vi "poly_control_value_from_name_multi.vi"(8 "error in (no error)":errorcluster, 9 "control names":string[](array[string]), 10 "vi ref":refnum<vi>) -> (0 "error out":errorcluster, 1 "Values":variant[](array[variant]), 2 "vi ref dup":refnum<vi>, 4 "found?":bool[](array[boolean]), 5 "ctrl refs":refnum<vi>[](array[refnum]))   [LabVIEW 2015]
uses:
  poly_control_ref_from_name_multi.vi
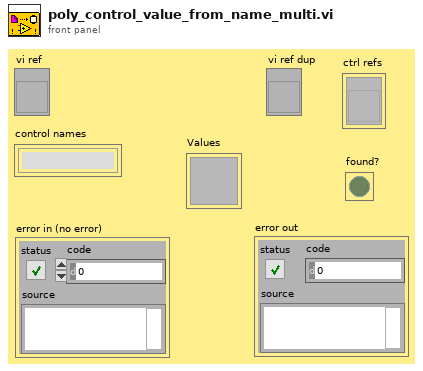
[diagram p1: front panel]
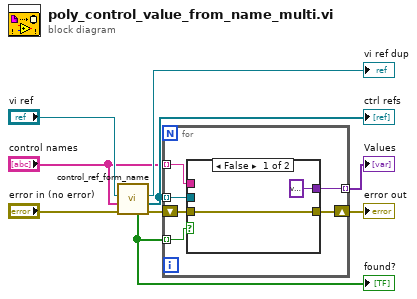
[diagram p0: block diagram]
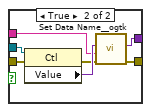
[diagram p2: hidden frame]
diagram:
  n1 = call-poly "control_ref_form_name.vi"("error in (no error)"="error in (no error)", "control names"="control names", "vi ref"="vi ref") -> ("error out"=w6:errorcluster, "ctrl refs"=w2:refnum<vi>[], "vi ref dup"=→"vi ref dup":refnum<vi>, "found?"=w3:bool[])  [unwired: 5 in]
  "ctrl refs" <- w2
  "found?" <- w3
  n2 = for {
    shift-right: [w14] -> w5
    shift-left: w6 -> [w15]
    tunnel: [w13] -> w4 mode=indexing
    tunnel: w3 -> [w12] mode=indexing
    tunnel: w2 -> [w11] mode=indexing
    tunnel: "control names" -> [w10] mode=indexing
    n3 = case shown="False" w12 {
      tunnel: w15 -> [w16 w24]
      tunnel: [w16 w19] -> w14
      tunnel: [variant w21] -> w13
      tunnel: w11 -> [_ w23]
      tunnel: w10 -> [_ w20]
      frame False {
      }
      frame True {
        n4 = property class="Ctl"(reference=w23, error in=w24) -> (error out=w18:errorcluster, "Value"=w22:variant)  [unwired: 1 out]
        n5 = call <userlib>:"Set Data Name__ogtk.vi"("error in (no error)"=w18, "Data Name"=w20, "Data"=w22) -> ("error out"=w19:errorcluster, "Renamed Data"=w21:variant)  [unwired: 7 in]
      }
    }
  }
  "error out" <- w5
  "Values" <- w4
